vi "Instantiate LV Dev.vi"   [LabVIEW 2019, in "LV DEV.lvclass"]
uses:
  LV DEV.lvclass
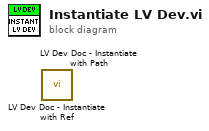
[diagram p0: block diagram]
diagram:
  n1 = call "LV Dev Doc - Instantiate with Ref.vi"() -> ()  [unwired: 14 in, 2 out]
  n2 = call "LV Dev Doc - Instantiate with Path.vi"() -> ()  [unwired: 14 in, 2 out]
